vi "clearStim.vi"(8 "error in (no error)":errorcluster, 11 "Stim in":refnum<class "Stim.lvclass">) -> (0 "error out":errorcluster, 3 "Stim out":refnum<class "Stim.lvclass">)   [LabVIEW 2014, in "Stim.lvclass"]
uses:
  Stim.lvclass
  Stim.lvclass/Stim.ctl
  <vilib>/DAQmx/write.llb/DAQmx Write.vi
  <vilib>/DAQmx/write.llb/DAQmx Write (Digital 1D Bool NChan 1Samp 1Line).vi
  <vilib>/DAQmx/miscellaneous.llb/DAQmx Fill In Error Info.vi
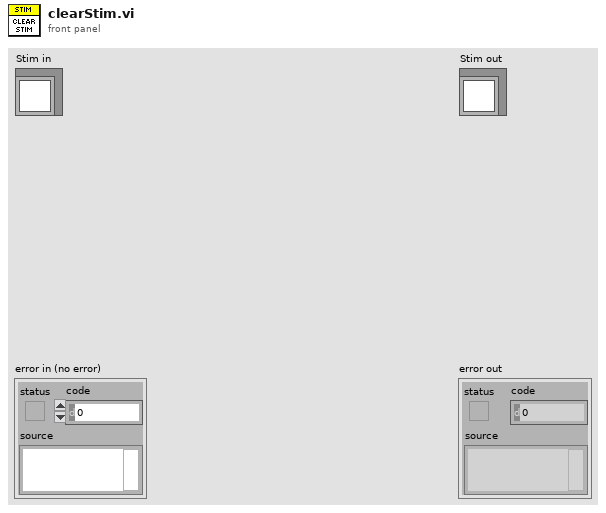
[diagram p1: front panel]
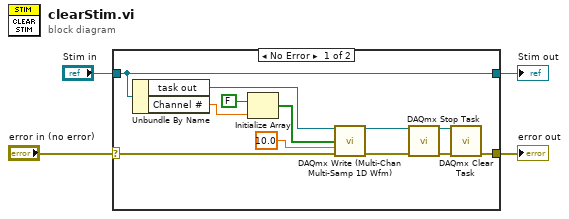
[diagram p0: block diagram]
diagram:
  n1 = case shown="No Error" "error in (no error)" {
    selector: "error in (no error)" -> [w9 w18]
    tunnel: [w13 w18] -> w1
    tunnel: [w16 w17] -> w2
    tunnel: "Stim in" -> [w16 w17]
    frame No Error {
      n2 = Unbundle By Name(w16) -> ("task out"=w10:refnum<k21>, "Channel #"=w6:dbl)
      n3 = Initialize Array(FALSE, w6) -> (w5:bool[])
      n4 = call-poly "DAQmx Write (Multi-Chan Multi-Samp 1D Wfm).vi"("task/channels in"=w10, "data"=w5, "timeout"=10.0, "error in"=w9) -> ("task out"=w11:refnum<k21>, "error out"=w8:errorcluster)  [unwired: 9 in, 1 out]
      n5 = call <vilib>:"DAQmx Stop Task.vi"("task/channels in"=w11, "error in"=w8) -> ("task out"=w15:refnum<k21>, "error out"=w14:errorcluster)  [unwired: 12 in]
      n6 = call <vilib>:"DAQmx Clear Task.vi"("task in"=w15, "error in"=w14) -> ("error out"=w13:errorcluster)  [unwired: 13 in]
    }
    frame Error {
    }
  }
  "error out" <- w1
  "Stim out" <- w2
